vi "PAQmem_initialize_database.vi"(8 "error in (no error)":errorcluster, 10 "Init_DB":T1, 11 "PAQ-memory in":refnum<class "PAQ-memory.lvclass">) -> (0 "error out":errorcluster, 2 "PAQ init string":string, 3 "PAQ-memory out":refnum<class "PAQ-memory.lvclass">)   [LabVIEW 2020, in "Sgraph_lib_V1.lvlib" / "PAQ-memory.lvclass"]
doc: "Andre Koelewijn, 27 feb 2021\nFrom one PAQ layer get initial data from disk during FAMM initialization"
uses:
  PAQ-memory.lvclass
  controls/PAQ_init.ctl
  PAQ-memory.lvclass/PAQ-memory.ctl
panel:
  out "appended path":path
  out "String":string
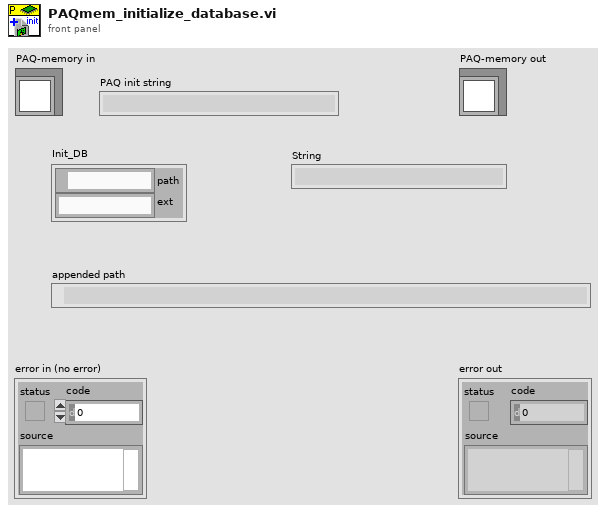
[diagram p1: front panel]
types:
  T1 = typedef "Sgraph_lib_V1.lvlib/PAQ-memory.lvclass/PAQ_init.ctl" = cluster{"path":path, "ext":string}
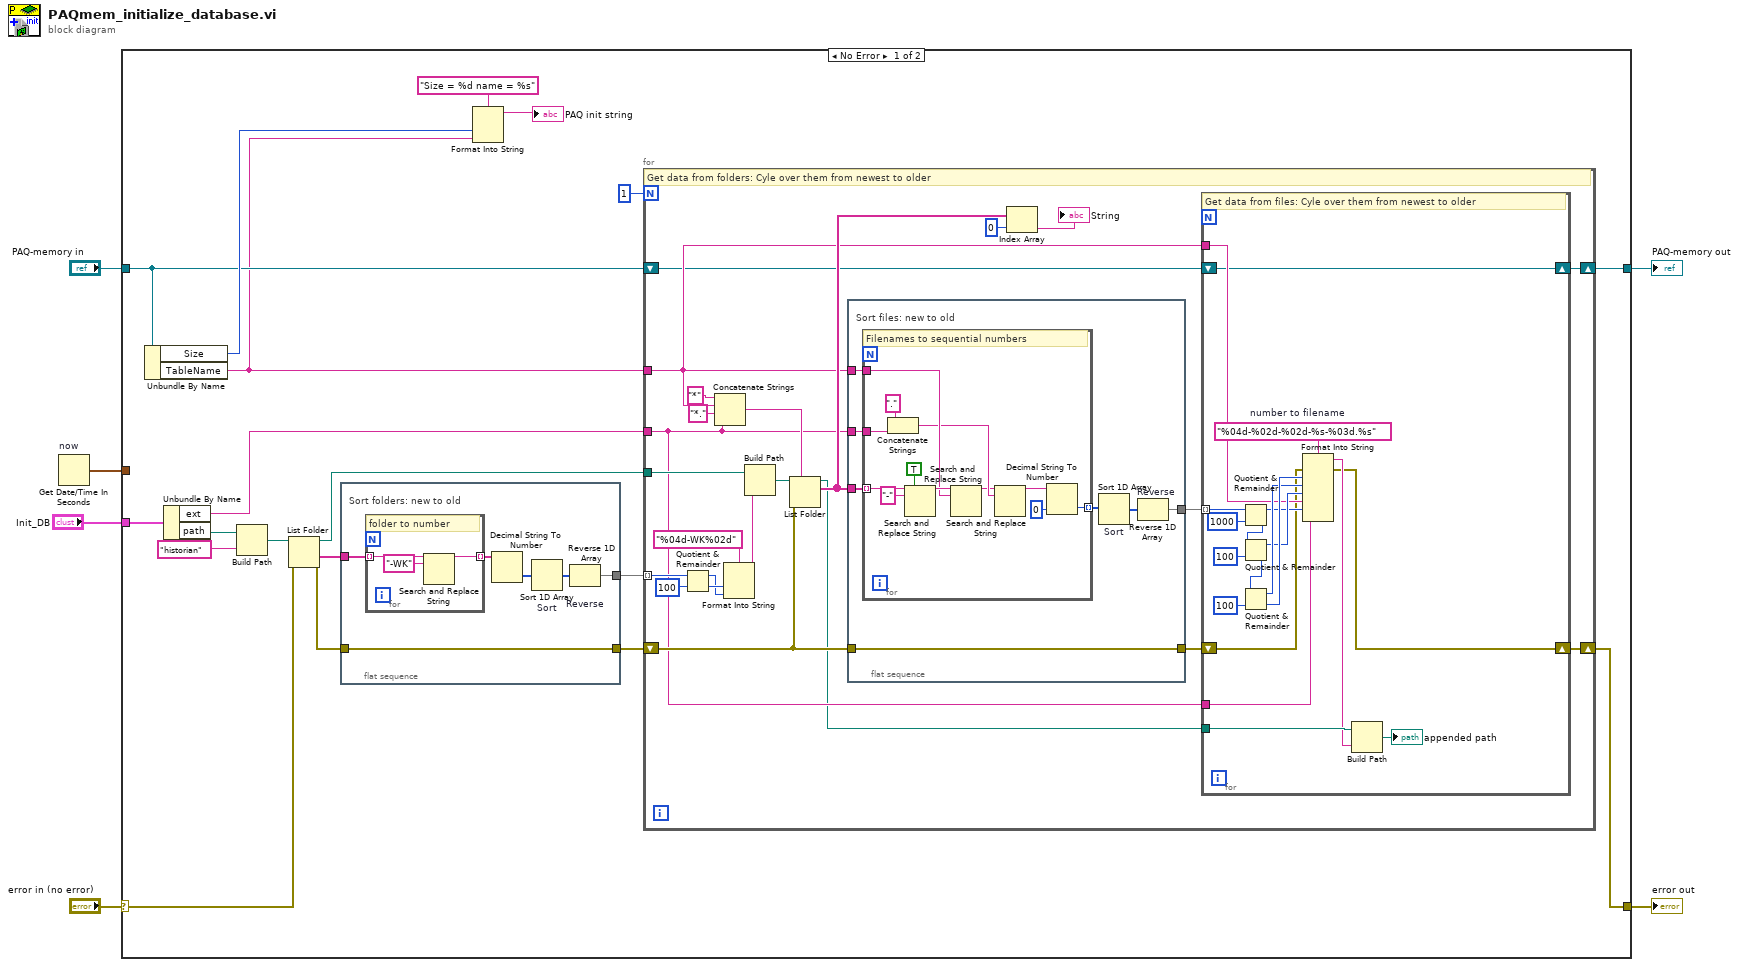
[diagram p0: block diagram]
diagram:
  n1 = Get Date/Time In Seconds "now"() -> (seconds since 1Jan1904=w2:timestamp)
  n2 = case shown="No Error" "error in (no error)" {
    selector: "error in (no error)" -> [w18 w97]
    tunnel: [w15 w97] -> w5
    tunnel: [w13 w96] -> w3
    tunnel: "PAQ-memory in" -> [w12 w96]
    tunnel: w2 -> [_ _]
    tunnel: "Init_DB" -> [w25 _]
    frame No Error {
      n3 = Unbundle By Name(w12) -> ("Size"=w20:i32, "TableName"=w8:string)
      n4 = Unbundle By Name(w25) -> ("ext"=w7:string, "path"=w24:path)
      n5 = Build Path(base path=w24, name or relative path="historian" ("string")) -> (appended path=w19:path)
      n6 = List Folder(path=w19, error in=w18) -> (path out=w9:path, folder names=w17:string[], error out=w16:errorcluster)  [unwired: 2 in, 1 out]
      n7 = flat-sequence {
        tunnel: w17 -> [w92]
        tunnel: [w87] -> w11
        tunnel: w16 -> [w89]
        tunnel: [w89] -> w14
        frame #0 {
          # "Sort folders: new to old"
          n8 = for {
            tunnel: w92 -> [w95] mode=indexing
            tunnel: [w93] -> w91 mode=indexing
            # "folder to number"
            n9 = Search and Replace String(input string=w95, search string="-WK") -> (result string=w93:string)  [unwired: 6 in, 3 out]
          }
          n10 = Decimal String To Number ("to num")(string=w91) -> (number=w90:i32[])  [unwired: 2 in, 1 out]
          n11 = Sort 1D Array "Sort"(array=w90) -> (sorted array=w88:i32[])
          n12 = Reverse 1D Array "Reverse"(array=w88) -> (reversed array=w87:i32[])
        }
      }
      n13 = Format Into String(format string="Size = %d name = %s", w20, w8) -> (resulting string=→"PAQ init string":string)  [unwired: 2 in, 1 out]
      n14 = for {
        N: 1 -> [_]
        shift-right: [w28] -> w15
        shift-left: w14 -> [w37]
        shift-right: [w26] -> w13
        shift-left: w12 -> [w27]
        tunnel: w11 -> [w48] mode=indexing
        tunnel: w7 -> [w31]
        tunnel: w9 -> [w43]
        tunnel: w8 -> [w32]
        # "Get data from folders: Cyle over them from newest to older"
        n15 = Quotient & Remainder(x=w48, y=100) -> (x-y*floor(x/y)=w44:i32, floor(x/y)=w45:i32)
        n16 = Concatenate Strings("*", w32, "*.", w31) -> (w38:string)
        n17 = Format Into String(format string="%04d-WK%02d", w45, w44) -> (resulting string=w42:string)  [unwired: 2 in, 1 out]
        n18 = Build Path(base path=w43, name or relative path=w42) -> (appended path=w41:path)
        n19 = List Folder(path=w41, pattern=w38, error in=w37) -> (path out=w30:path, filenames=w35:string[])  [unwired: 1 in, 2 out]
        n20 = flat-sequence {
          tunnel: w35 -> [w74]
          tunnel: w32 -> [w73]
          tunnel: w31 -> [w72]
          tunnel: [w69] -> w36
          tunnel: w37 -> [w68]
          tunnel: [w68] -> w29
          frame #0 {
            # "Sort files: new to old"
            n21 = for {
              tunnel: w74 -> [w75] mode=indexing
              tunnel: w73 -> [w83]
              tunnel: w72 -> [w82]
              tunnel: [w77] -> w70 mode=indexing
              # "Filenames to sequential numbers"
              n22 = Concatenate Strings("." ("string"), w82) -> (w81:string)
              n23 = Search and Replace String(replace all?=TRUE ("replace all? (F)"), input string=w75, search string="-") -> (result string=w84:string)  [unwired: 5 in, 3 out]
              n24 = Search and Replace String(input string=w84, search string=w83) -> (result string=w80:string)  [unwired: 6 in, 3 out]
              n25 = Search and Replace String(input string=w80, search string=w81) -> (result string=w78:string)  [unwired: 6 in, 3 out]
              n26 = Decimal String To Number(string=w78, default (0L)=u64 0 ("default (0 I32)")) -> (number=w77:u64)  [unwired: 1 in, 1 out]
            }
            n27 = Sort 1D Array "Sort"(array=w70) -> (sorted array=w71:u64[])
            n28 = Reverse 1D Array "Reverse"(array=w71) -> (reversed array=w69:u64[])
          }
        }
        n29 = Index Array(array=w35, index=0) -> (element=→"String":string)
        n30 = for {
          tunnel: w36 -> [w66] mode=indexing
          tunnel: w32 -> [w57]
          tunnel: w31 -> [w55]
          tunnel: w30 -> [w54]
          shift-right: [w51] -> w28
          shift-left: w29 -> [w52]
          shift-right: [w49] -> w26
          shift-left: w27 -> [w49]
          w61 = "%04d-%02d-%02d-%s-%03d.%s"  # number to filename
          # "Get data from files: Cyle over them from newest to older"
          n31 = Quotient & Remainder(x=w66, y=u64 1000) -> (x-y*floor(x/y)=w56:u64, floor(x/y)=w64:u64)
          n32 = Quotient & Remainder(x=w64, y=u64 100) -> (x-y*floor(x/y)=w58:u64, floor(x/y)=w62:u64)
          n33 = Quotient & Remainder(x=w62, y=u64 100) -> (x-y*floor(x/y)=w59:u64, floor(x/y)=w60:u64)
          n34 = Format Into String(format string=w61, error in=w52, w60, w59, w58, w57, w56, w55) -> (resulting string=w53:string, error out=w51:errorcluster)  [unwired: 1 in]
          n35 = Build Path(base path=w54, name or relative path=w53) -> (appended path=→"appended path":path)
        }
      }
    }
    frame Error {
    }
  }
  "error out" <- w5
  "PAQ-memory out" <- w3
